vi "Find contact point.vi"(0 "reference in":refnum<class "Fcurve.lvclass">, 2 "Z pos (V)":dbl[](array[numeric]), 5 "error in (no error)":errorcluster) -> (14 "reference out":refnum<class "Fcurve.lvclass">, 16 "contact index":i32, 19 "error out":errorcluster)   [LabVIEW 2019, in "Fcurve.lvclass"]
uses:
  Fcurve.lvclass
panel:
  out "Fcurve Metadata.Zpos contact":dbl
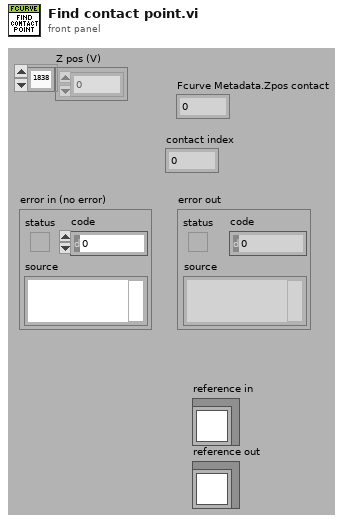
[diagram p1: front panel]
types:
  T1 = typedef "Fcurve.lvclass/ObjectAttributes.ctl" = cluster{"MyAttribute":dbl, "Fcurve Metadata":T2, "Contact Spread of dev":dbl, "Tau Delay (ms)":dbl, "Points of contact":dbl, "Def_wfm":cluster{"Max":dbl, "Min":dbl}, "Zpos_wfm":cluster{"Max":dbl, "Min":dbl}, "Contact stat?":bool, "Real AI dt (s)":dbl, "Decimation":cluster{"App":cluster{"Dec":i32, "apply":bool}, "Con":cluster{"Dec":i32, "apply":bool}, "Ret":cluster{"Dec":i32, "apply":bool}}, "Segment def[0]":dbl, "Segment Zpos[0]":dbl, "Raw Datum":waveform(dbl)[], "Group metadata":T3, "M_data obj":refnum<class "metadata.lvclass">, "Channel name(s)":string[], "Segment fcurve data":cluster{"X":dbl[], "Y":dbl[]}[], "Segment duration":cluster{"Start":i32, "Duration":i32}[], "Segment info":T4[], "Segment durations (S)":dbl[], "Segments Maxmin":T6[]}
  T2 = typedef "Fcurve.lvclass/Metadata.ctl" = cluster{"dt (us)":dbl, "Dec Factor":dbl, "Z piezo Sensitivity (nm/V)":dbl, "K (N/m)":dbl, "Sp (V)":dbl, "Contact (ms)":dbl, "Zpos contact":dbl, "Vel_app (nm/s)":dbl, "Vel_ret (nm/s)":dbl, "deltaV (nm)":dbl, "Def_V0 (v)":dbl, "Piezo gain":dbl, "invOLS (nm/V)":dbl}
  T3 = typedef "TDMS_DataHandler.lvclass/Fcurve Meta data.ctl" = cluster{"property names":string[], "property values":variant[]}
  T4 = typedef "Fcurve.lvclass/Fcurve segments --cluster.ctl" = cluster{"type":T5, "nb points":i32, "dec factor":u32, "sampling rate (S/s)":u32}
  T5 = typedef "metadata.lvclass/Segment type--combobox.ctl" = string
  T6 = typedef "Fcurve.lvclass/Segment MaxMin --cluster.ctl" = cluster{"Def":cluster{"max value":dbl, "min value":dbl}, "Zpos":cluster{"max value":dbl, "min value":dbl}}
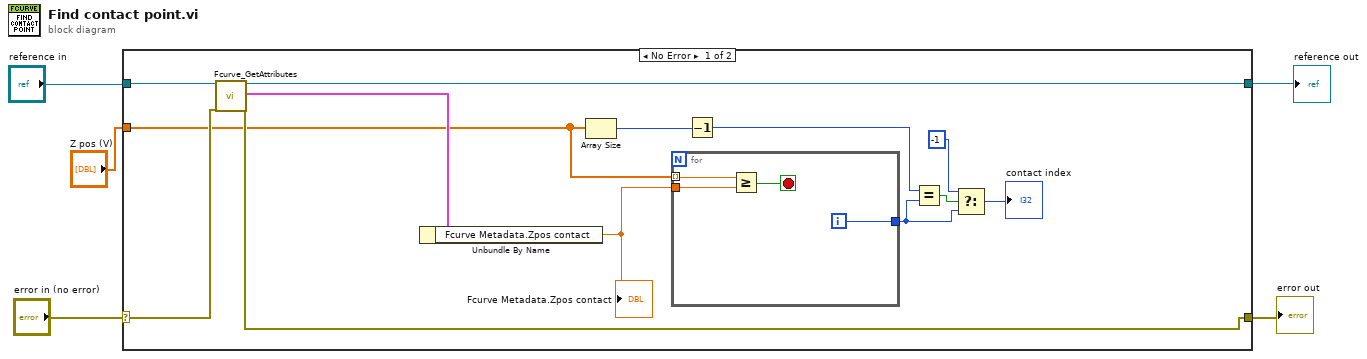
[diagram p0: block diagram]
diagram:
  n1 = case shown="No Error" "error in (no error)" {
    selector: "error in (no error)" -> [w12 w24]
    tunnel: [w8 w24] -> w4
    tunnel: "reference in" -> [w11 w23]
    tunnel: [w6 w23] -> w2
    tunnel: "Z pos (V)" -> [w7 _]
    frame No Error {
      n2 = call "Fcurve_GetAttributes.vi"("reference in"=w11, "error in (no error)"=w12) -> ("reference out"=w6:refnum<class "Fcurve.lvclass">, "attributes"=w10:T1, "error out"=w8:errorcluster)  [unwired: 14 in, 1 out]
      n3 = Unbundle By Name(w10) -> ("Fcurve Metadata.Zpos contact"=w9:dbl)
      "Fcurve Metadata.Zpos contact" <- w9
      n4 = Array Size(array=w7) -> (size(s)=w18:i32)
      n5 = for {
        tunnel: w7 -> [w22] mode=indexing
        tunnel: w9 -> [w21]
        tunnel: [w19] -> w15
        i -> [w19]
        stop <- w20 stop-if-true
        n6 = Greater Or Equal?(x=w22, y=w21) -> (x >= y?=w20:bool)
      }
      n7 = Decrement(x=w18) -> (x-1=w17:i32)
      n8 = Equal?(x=w17, y=w15) -> (x = y?=w16:bool)
      n9 = Select(t=-1, s=w16, f=w15) -> (s? t:f=→"contact index":i32)
    }
    frame Error {
    }
  }
  "error out" <- w4
  "reference out" <- w2
